vi "Queue Key Down.vi"(6 "Queue Ref Out":T1, 7 "C":i16, 8 "error in (no error)":errorcluster caption="Error In", 9 "Platform Key":T2, 10 "Group Key":cluster{"Num Pad":bool, "Menu Key":bool}, 11 "V Key":T3 caption="V键") -> (0 "error out":errorcluster caption="Error Out")   [LabVIEW 2020]
uses:
  <vilib>/event_ctls.llb/eventvkey.ctl
  000 Module Data Type.ctl
  Queue Message.ctl
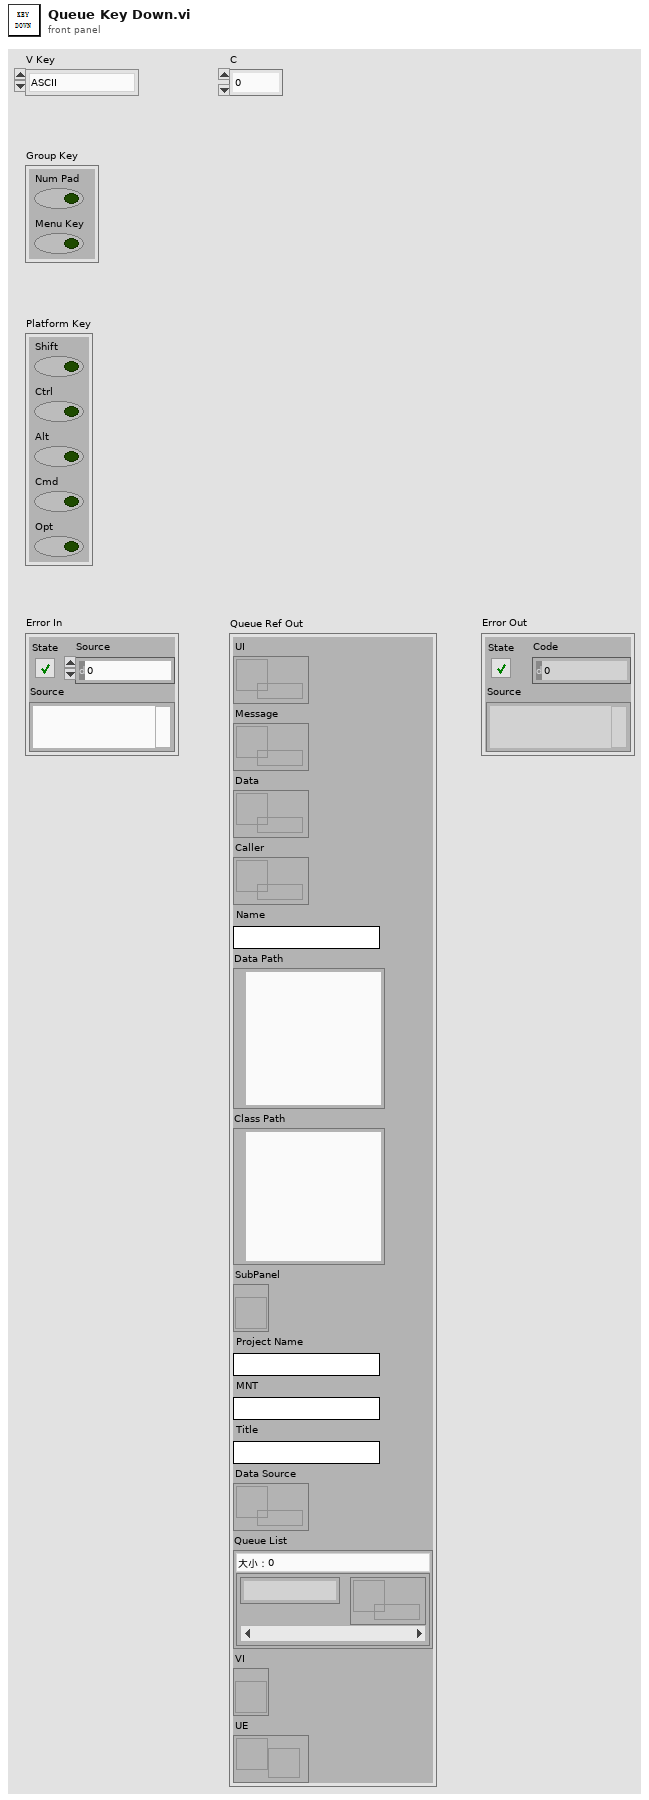
[diagram p1: front panel]
types:
  T1 = typedef "000 Module Data Type.ctl" = cluster{"UI":refnum<queue>, "Message":refnum<queue>, "Data":refnum<queue>, "Caller":refnum<queue>, "Name":string, "Data Path":path, "Class Path":path, "SubPanel":refnum<vi>, "Project Name":string, "MNT":string, "Title":string, "Data Source":refnum<queue>, "Queue List":map{string, refnum<queue>}, "VI":refnum<vi>, "UE":refnum<user-event>}
  T2 = cluster{"Shift":bool, "Ctrl":bool, "Alt":bool, "Cmd":bool, "Opt":bool}
  T3 = typedef "eventvkey.ctl" = enum16{"ASCII", "Enter", "Return", "Shift", "Ctrl", "Alt", "Cmd", "Opt", "Caps", "NumLock", "Clear", "Break", "Up", "Down", "Left", "Right", "Insert", "Delete", "Home", "End", "PageUp", "PageDown", "Escape", "Help", "Pause", "ScrollLock", "F1", "F2", "F3", "F4", "F5", "F6", "F7", "F8", "F9", "F10", "F11", "F12", "F13", "F14", "F15", "F16", "F17", "F18", "F19", "F20", "F21", "F22", "F23", "F24", "Play", "VolumeUp", "VolumeDown", "Mute", "Two Byte Char"}
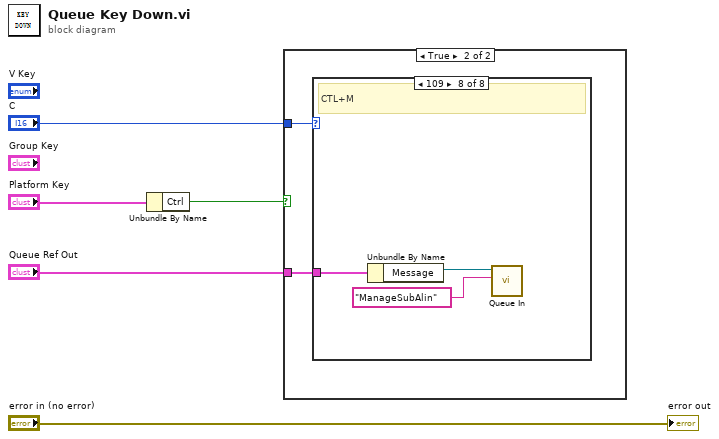
[diagram p0: block diagram]
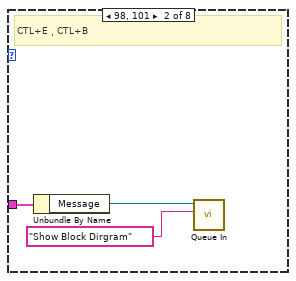
[diagram p4: hidden frame]
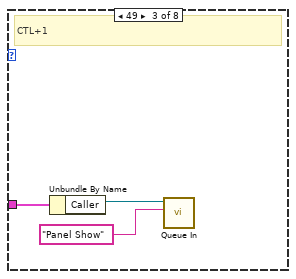
[diagram p5: hidden frame]
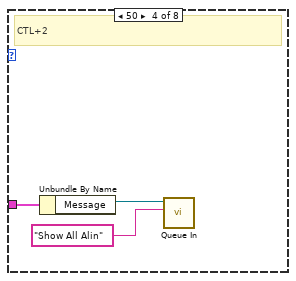
[diagram p6: hidden frame]
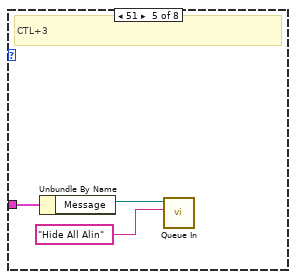
[diagram p7: hidden frame]
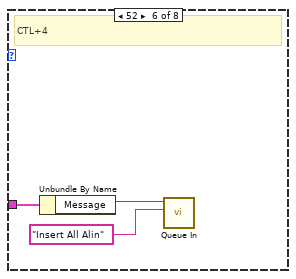
[diagram p8: hidden frame]
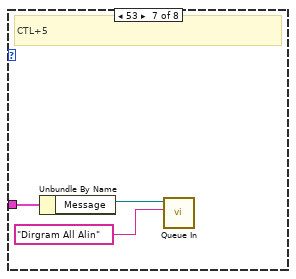
[diagram p9: hidden frame]
diagram:
  n1 = Unbundle By Name("Platform Key") -> ("Ctrl"=w3:bool)
  n2 = case shown="True" w3 {
    tunnel: "C" -> [_ w7]
    tunnel: "Queue Ref Out" -> [_ w6]
    frame False {
    }
    frame True {
      n3 = case shown="109" w7 {
        tunnel: w6 -> [_ w9 w11 w14 w17 w20 w23 w26]
        frame 0, Default {
        }
        frame 98, 101 {
          # "CTL+E，CTL+B"
          n4 = Unbundle By Name(w9) -> ("Message"=w8:refnum<queue>)
          n5 = call "Queue In.vi"("Message"="Show Block Dirgram", "Queue In"=w8) -> ()  [unwired: 8 in, 2 out]
        }
        frame 49 {
          # "CTL+1"
          n6 = Unbundle By Name(w11) -> ("Caller"=w13:refnum<queue>)
          n7 = call "Queue In.vi"("Message"="Panel Show", "Queue In"=w13) -> ()  [unwired: 8 in, 2 out]
        }
        frame 50 {
          # "CTL+2"
          n8 = Unbundle By Name(w14) -> ("Message"=w16:refnum<queue>)
          n9 = call "Queue In.vi"("Message"="Show All Alin", "Queue In"=w16) -> ()  [unwired: 8 in, 2 out]
        }
        frame 51 {
          # "CTL+3"
          n10 = Unbundle By Name(w17) -> ("Message"=w19:refnum<queue>)
          n11 = call "Queue In.vi"("Message"="Hide All Alin", "Queue In"=w19) -> ()  [unwired: 8 in, 2 out]
        }
        frame 52 {
          # "CTL+4"
          n12 = Unbundle By Name(w20) -> ("Message"=w22:refnum<queue>)
          n13 = call "Queue In.vi"("Message"="Insert All Alin", "Queue In"=w22) -> ()  [unwired: 8 in, 2 out]
        }
        frame 53 {
          # "CTL+5"
          n14 = Unbundle By Name(w23) -> ("Message"=w25:refnum<queue>)
          n15 = call "Queue In.vi"("Message"="Dirgram All Alin", "Queue In"=w25) -> ()  [unwired: 8 in, 2 out]
        }
        frame 109 {
          # "CTL+M"
          n16 = Unbundle By Name(w26) -> ("Message"=w28:refnum<queue>)
          n17 = call "Queue In.vi"("Message"="ManageSubAlin", "Queue In"=w28) -> ()  [unwired: 8 in, 2 out]
        }
      }
    }
  }
  "error out" <- "error in (no error)"
